vi "AutoProgramState.vi"(3 "error in (no error)":errorcluster, 4 "INcluster":T2, 6 "G-Code Array":string[](array[string])) -> (0 "error in (no error) 2":errorcluster, 1 "Stop State":bool, 2 "Next Command":string)   [LabVIEW 2017, in "LibraryGcode.lvlib"]
uses:
  LibraryGcode.lvlib
  control/Queue/QueueCMDandPOS.ctl
  control/Queue/TypeDataPOS.ctl
  control/stateCmdUpdatePara.ctl
  ClassStateAuto/StateMachine_Auto.ctl
  ClassStateAuto/StateAuto.lvclass
  variableGlobal/StartAutoandGcode.vi
panel:
  out "Enum":T1
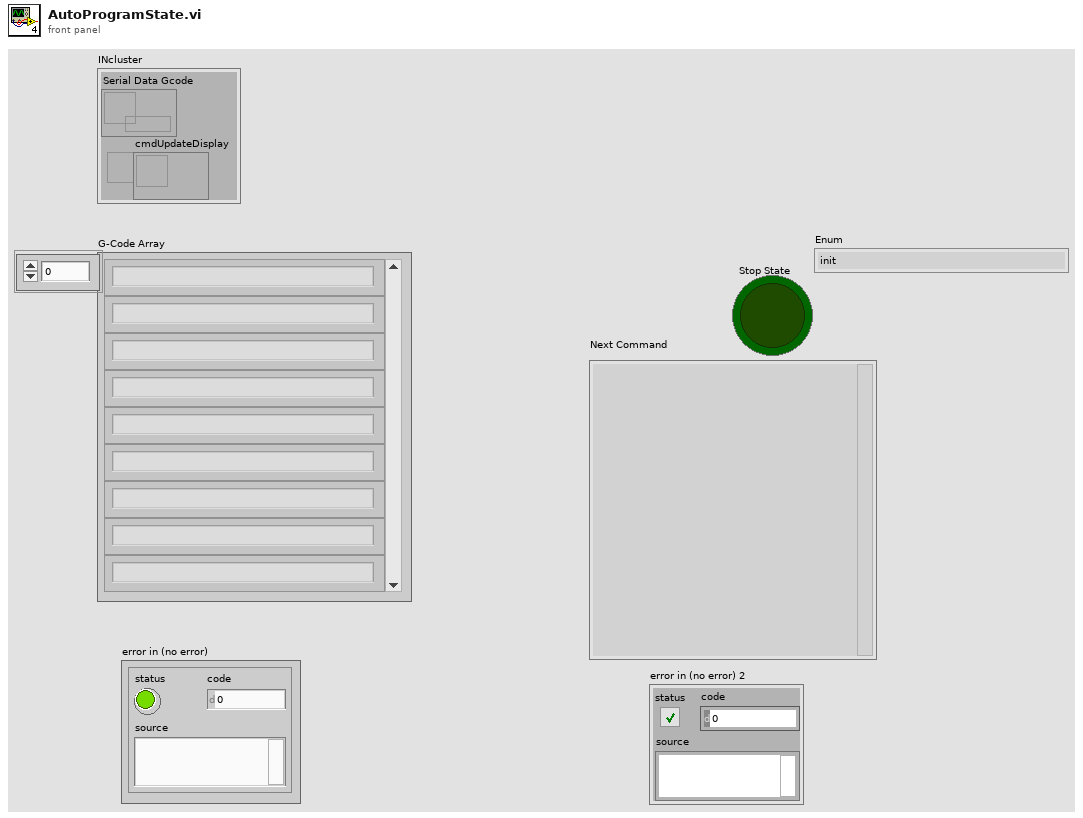
[diagram p1: front panel]
types:
  T1 = typedef "LibraryGcode.lvlib/StateAuto.lvclass/StateMachine_Auto.ctl" = enum16{"init", "checkEMG", "checkStateBoard", "checkQueue", "writeDataQueue", "WaitToRunning", "initNextCommand", "endNextCommand"}
  T2 = typedef "LibraryGcode.lvlib/QueueCMDandPOS.ctl" = cluster{"Serial Data Gcode":refnum<queue>, "cmdUpdateDisplay":refnum<queue>}
  T3 = typedef "LibraryGcode.lvlib/stateBoardFirmware.ctl" = enum16{"Running", "Waiting", "Pos", "IDLE"}
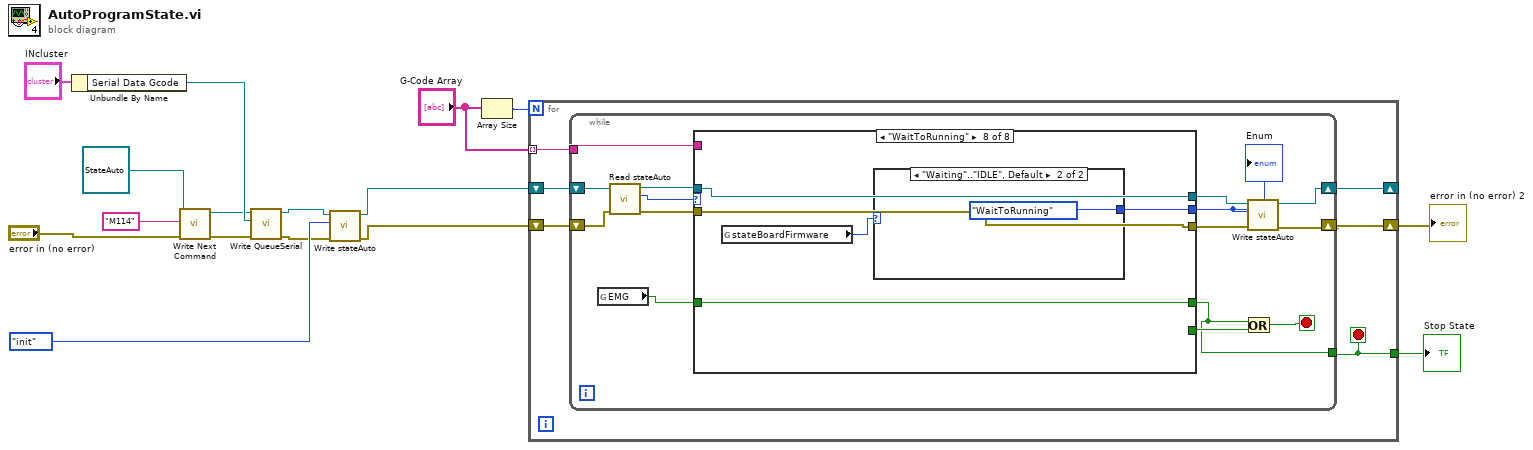
[diagram p0: block diagram]
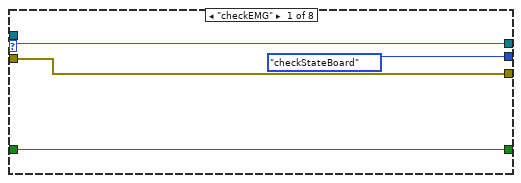
[diagram p2: hidden frame]
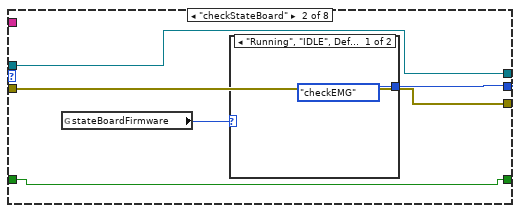
[diagram p3: hidden frame]
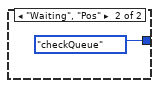
[diagram p4: hidden frame]
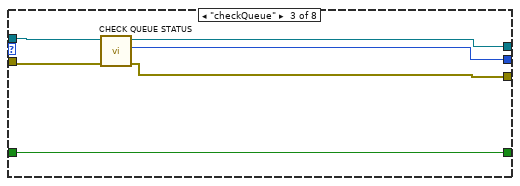
[diagram p5: hidden frame]
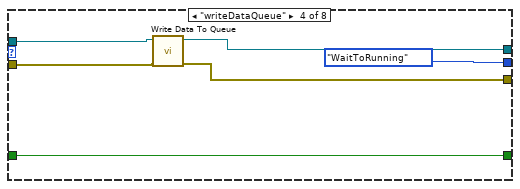
[diagram p6: hidden frame]
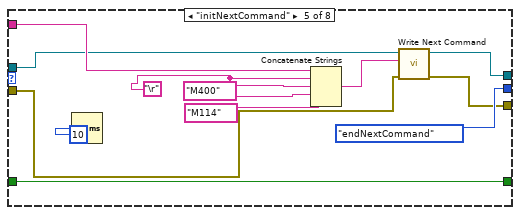
[diagram p7: hidden frame]
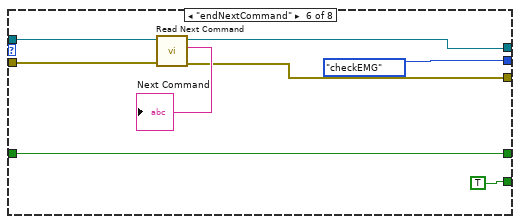
[diagram p8: hidden frame]
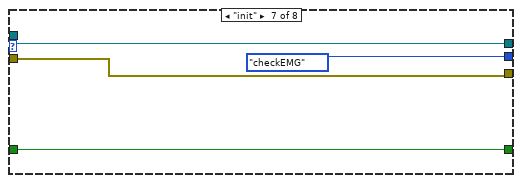
[diagram p9: hidden frame]
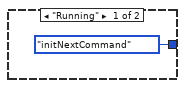
[diagram p10: hidden frame]
diagram:
  n1 = Unbundle By Name("INcluster") -> ("Serial Data Gcode"=w11:refnum<queue>)
  n2 = call-dynamic "Write Next Command.vi"("error in (no error)"="error in (no error)", "Next Command"="M114", "StateAuto in"=refnum<class "StateAuto.lvclass"> refnum) -> ("error out"=w5:errorcluster, "StateAuto out"=w9:refnum<class "StateAuto.lvclass">)  [unwired: 7 in]
  n3 = call-dynamic "Write QueueSerial.vi"("error in (no error)"=w5, "QueueSerial"=w11, "StateAuto in"=w9) -> ("error out"=w4:errorcluster, "StateAuto out"=w8:refnum<class "StateAuto.lvclass">)  [unwired: 7 in]
  n4 = call-dynamic "Write stateAuto.vi"("error in (no error)"=w4, "Enum"=StateMachine_Auto."init", "StateAuto in"=w8) -> ("error out"=w3:errorcluster, "StateAuto out"=w7:refnum<class "StateAuto.lvclass">)  [unwired: 7 in]
  n5 = Array Size(array="G-Code Array") -> (size(s)=w15:i32)
  n6 = for {
    N: w15 -> [_]
    tunnel: "G-Code Array" -> [w22] mode=indexing
    tunnel: [w21] -> w13
    shift-right: [w19] -> _
    shift-left: w7 -> [w20]
    shift-right: [w17] -> w1
    shift-left: w3 -> [w18]
    stop <- w21 stop-if-true
    n7 = while {
      tunnel: w22 -> [w37]
      tunnel: [w24] -> w21
      shift-right: [w25] -> w19
      shift-left: w20 -> [w34]
      shift-right: [w29] -> w17
      shift-left: w18 -> [w30]
      stop <- w36 stop-if-true
      n8 = global read "StartAutoandGcode.vi" "EMG"() -> (w23:bool)
      n9 = call-dynamic "Read stateAuto.vi"("error in (no error)"=w30, "StateAuto in"=w34) -> ("error out"=w26:errorcluster, "Enum"=w32:T1, "StateAuto out"=w33:refnum<class "StateAuto.lvclass">)  [unwired: 7 in]
      n10 = case shown="\"WaitToRunning\"" w32 {
        tunnel: w37 -> [_ _ _ _ w70 _ _ _]
        tunnel: [_ _ _ _ _ TRUE ("y") _ _] -> w35
        tunnel: [w39 w44 w52 w57 w64 w75 w82 w88] -> w28
        tunnel: w33 -> [w41 w43 w54 w59 w65 w79 w84 w89]
        tunnel: [w41 w43 w51 w55 w63 w74 w84 w89] -> w31
        tunnel: [StateMachine_Auto."checkStateBoard" ("Enum") w45 w50 StateMachine_Auto."WaitToRunning" ("Enum") StateMachine_Auto."endNextCommand" ("Enum") StateMachine_Auto."checkEMG" ("Enum") StateMachine_Auto."checkEMG" ("Enum") w87] -> w27
        tunnel: w26 -> [w39 w44 w53 w58 w62 w76 w82 w88]
        tunnel: w23 -> [w38 w42 w49 w56 w61 w73 w81 w86]
        tunnel: [w38 w42 w49 w56 w61 w73 w81 w86] -> w24
        frame "checkEMG" {
        }
        frame "checkStateBoard" {
          n11 = global read "StartAutoandGcode.vi" "stateBoardFirmware"() -> (w46:T3)
          n12 = case shown="\"Running\", \"IDLE\", Default" w46 {
            tunnel: [StateMachine_Auto."checkEMG" ("Enum") StateMachine_Auto."checkQueue" ("Enum")] -> w45
            frame "Running", "IDLE", Default {
            }
            frame "Waiting", "Pos" {
            }
          }
        }
        frame "checkQueue" {
          n13 = call-dynamic "CHECK QUEUE STATUS.vi"("error in (no error)"=w53, "StateAuto in"=w54) -> ("error out"=w52:errorcluster, "stateAuto"=w50:T1, "StateAuto out"=w51:refnum<class "StateAuto.lvclass">)  [unwired: 7 in]
        }
        frame "writeDataQueue" {
          n14 = call-dynamic "Write Data To Queue.vi"("error in (no error)"=w58, "StateAuto in"=w59) -> ("error out"=w57:errorcluster, "StateAuto out"=w55:refnum<class "StateAuto.lvclass">)  [unwired: 8 in]
        }
        frame "initNextCommand" {
          w69 = "\r"
          n15 = Wait (ms)(milliseconds to wait=u32 10) -> ()  [unwired: 1 out]
          n16 = Concatenate Strings(w70, w69, "M400" ("string"), w69, "M114" ("string")) -> (w67:string)
          n17 = call-dynamic "Write Next Command.vi"("error in (no error)"=w62, "Next Command"=w67, "StateAuto in"=w65) -> ("error out"=w64:errorcluster, "StateAuto out"=w63:refnum<class "StateAuto.lvclass">)  [unwired: 7 in]
        }
        frame "endNextCommand" {
          n18 = call-dynamic "Read Next Command.vi"("error in (no error)"=w76, "StateAuto in"=w79) -> ("error out"=w75:errorcluster, "Next Command"=→"Next Command":string, "StateAuto out"=w74:refnum<class "StateAuto.lvclass">)  [unwired: 7 in]
        }
        frame "init" {
        }
        frame "WaitToRunning" {
          n19 = global read "StartAutoandGcode.vi" "stateBoardFirmware"() -> (w85:T3)
          n20 = case shown="\"Waiting\"..\"IDLE\", Default" w85 {
            tunnel: [StateMachine_Auto."initNextCommand" ("Enum") StateMachine_Auto."WaitToRunning" ("Enum")] -> w87
            frame "Running" {
            }
            frame "Waiting".."IDLE", Default {
            }
          }
        }
      }
      "Enum" <- w27
      n21 = Or(x=w24, y=w35) -> (x .or. y?=w36:bool)
      n22 = call-dynamic "Write stateAuto.vi"("error in (no error)"=w28, "Enum"=w27, "StateAuto in"=w31) -> ("error out"=w29:errorcluster, "StateAuto out"=w25:refnum<class "StateAuto.lvclass">)  [unwired: 7 in]
    }
  }
  "Stop State" <- w13
  "error in (no error) 2" <- w1
